vi "SRV_Ain.vi"(0 "Variable Name":string="Sensor", 2 "SuperPro":T1, 3 "Channel":enum16{"1", "2", "3", "4", "5"}(ring)) -> (1 "Variable Out":string="WORK1", 4 "SuperPro":T1)   [LabVIEW 2009]
uses:
  <userlib>/SuperPro/OpCodes/_SubVIs/SuperProControl.ctl
panel:
  # "This LabVIEW item is deprecated.\n\nIt is believed to be unused and will be removed in a future version of SRV."
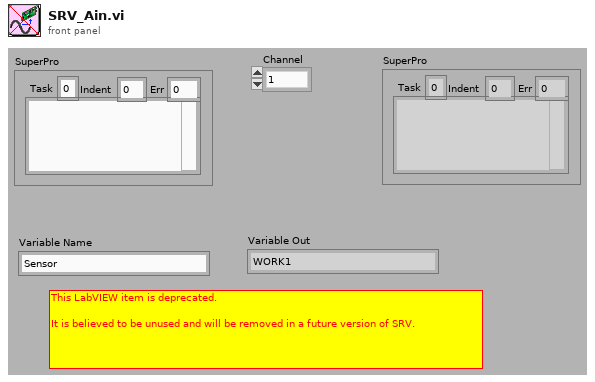
[diagram p1: front panel]
types:
  T1 = typedef "SuperProControl.ctl" = cluster{"Task":i32, "Indent":i32, "Err":i32, "ASM":string}
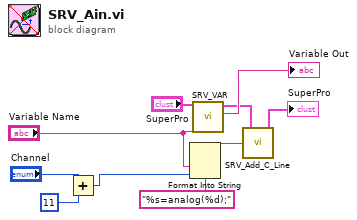
[diagram p0: block diagram]
diagram:
  n1 = Add(x="Channel", y=11) -> (x+y=w2:i32)
  n2 = Format Into String(format string="%s=analog(%d);", "Variable Name", w2) -> (resulting string=w8:string)  [unwired: 2 in, 1 out]
  n3 = call "SRV_VAR.vi"("SuperPro in"="SuperPro", "Name"="Variable Name") -> ("SuperPro out"=w4:T1, "Name"=→"Variable Out":string)  [unwired: 1 in, 2 out]
  n4 = call "SRV_Add_C_Line.vi"("C String"=w8, "SuperPro in"=w4) -> ("SuperPro out"=→"SuperPro":T1)  [unwired: 3 in]
